vi "Launcher.vi"() -> ()   [LabVIEW 2018]
panel:
  in  "Exit btn":bool
  in  "Script editor btn":bool
  in  "Results viewer btn":bool
  in  "Measurement mngr btn":bool
  in  "Instrument monitor btn":bool
  in  "Rapid-scanner btn":bool
  in  "Mapper btn":bool
  in  "FDMR btn":bool
  in  "CW-EPR btn":bool
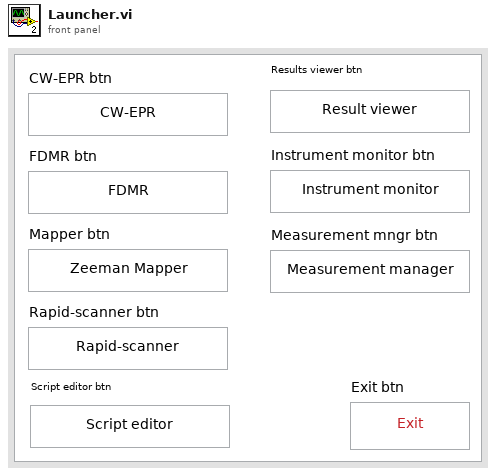
[diagram p1: front panel]
types:
  T1 = enum16{"Initialize", "Wait for event", "Run CW-EPR", "End CW-EPR", "Run FDMR", "End FDMR", "Run Mapper", "End Mapper", "Run Rapid-scanner", "End Rapid-scanner", "Run Script editor ", "End Script editor", "Run Results viewer", "End Result Viewer", "Show Instr mngr", "Hide Instr mngr", "Show meas mngr", "Hide meas mngr", "End All"}
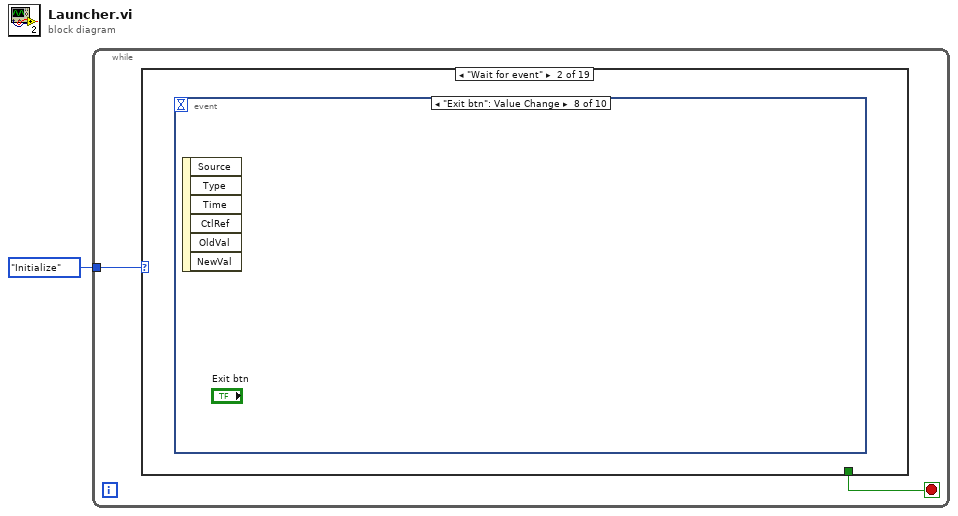
[diagram p0: block diagram]
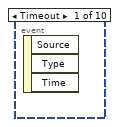
[diagram p3: hidden frame]
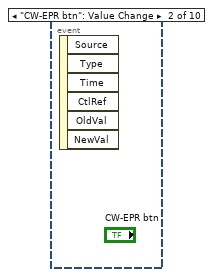
[diagram p4: hidden frame]
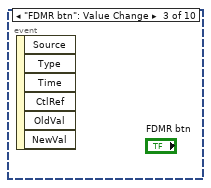
[diagram p5: hidden frame]
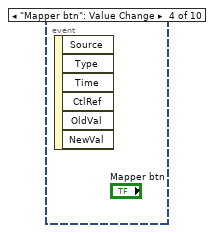
[diagram p6: hidden frame]
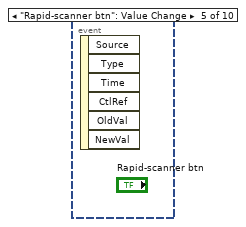
[diagram p7: hidden frame]
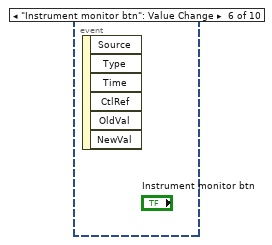
[diagram p8: hidden frame]
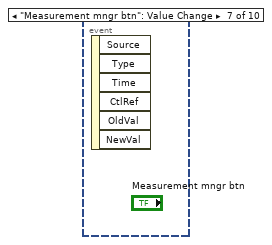
[diagram p9: hidden frame]
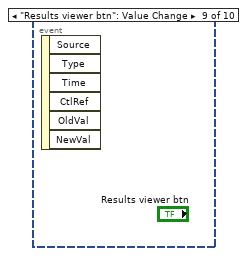
[diagram p10: hidden frame]
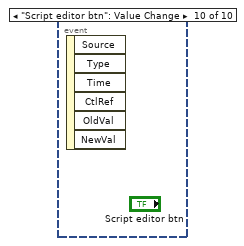
[diagram p11: hidden frame]
diagram:
  n1 = while {
    tunnel: T1."Initialize" -> [w3]
    stop <- w2 stop-if-true
    n2 = case shown="\"Wait for event\"" w3 {
      tunnel: [_ _ _ _ _ _ _ _ _ _ _ _ _ _ _ _ _ _ TRUE] -> w2
      frame "Initialize", Default {
      }
      frame "Wait for event" {
        n3 = event shown="[7] \"Exit btn\": Value Change" {
          selector: _ -> [_ _ _ _ _ _ _ _ _ _]
          dyn-events: _ -> [_ _ _ _ _ _ _ _ _ _]
          timeout: _ -> [_ _ _ _ _ _ _ _ _ _]
          event Timeout {
            n4 = event-data() -> ()  [unwired: 1 in, 3 out]
          }
          event "CW-EPR btn": Value Change {
            n5 = event-data() -> ()  [unwired: 1 in, 6 out]
          }
          event "FDMR btn": Value Change {
            n6 = event-data() -> ()  [unwired: 1 in, 6 out]
          }
          event "Mapper btn": Value Change {
            n7 = event-data() -> ()  [unwired: 1 in, 6 out]
          }
          event "Rapid-scanner btn": Value Change {
            n8 = event-data() -> ()  [unwired: 1 in, 6 out]
          }
          event "Instrument monitor btn": Value Change {
            n9 = event-data() -> ()  [unwired: 1 in, 6 out]
          }
          event "Measurement mngr btn": Value Change {
            n10 = event-data() -> ()  [unwired: 1 in, 6 out]
          }
          event "Exit btn": Value Change {
            n11 = event-data() -> ()  [unwired: 1 in, 6 out]
          }
          event "Results viewer btn": Value Change {
            n12 = event-data() -> ()  [unwired: 1 in, 6 out]
          }
          event "Script editor btn": Value Change {
            n13 = event-data() -> ()  [unwired: 1 in, 6 out]
          }
        }
      }
      frame "Run CW-EPR" {
      }
      frame "End CW-EPR" {
      }
      frame "Run FDMR" {
      }
      frame "End FDMR" {
      }
      frame "Run Mapper" {
      }
      frame "End Mapper" {
      }
      frame "Run Rapid-scanner" {
      }
      frame "End Rapid-scanner" {
      }
      frame "Run Script editor " {
      }
      frame "End Script editor" {
      }
      frame "Run Results viewer" {
      }
      frame "End Result Viewer" {
      }
      frame "Show Instr mngr" {
      }
      frame "Hide Instr mngr" {
      }
      frame "Show meas mngr" {
      }
      frame "Hide meas mngr" {
      }
      frame "End All" {
      }
    }
  }
